vi "油动机输入合法性检查.vi"(3 "error in (no error)":errorcluster) -> (0 "error out":errorcluster, 2 "油动机名称":string)   [LabVIEW 2013]
panel:
  in  "油动机名称库":string[](array[string])
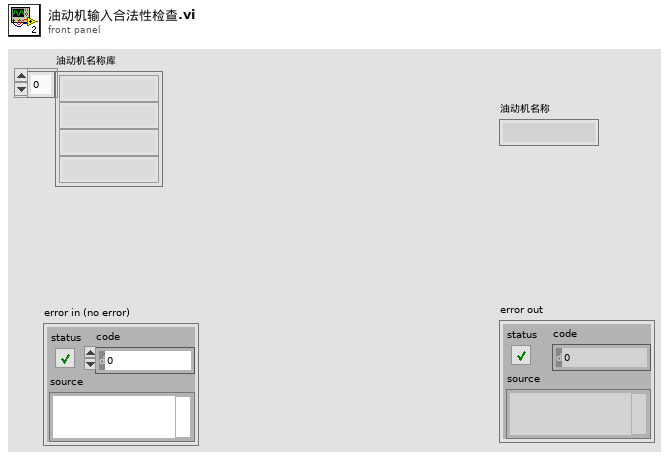
[diagram p1: front panel]
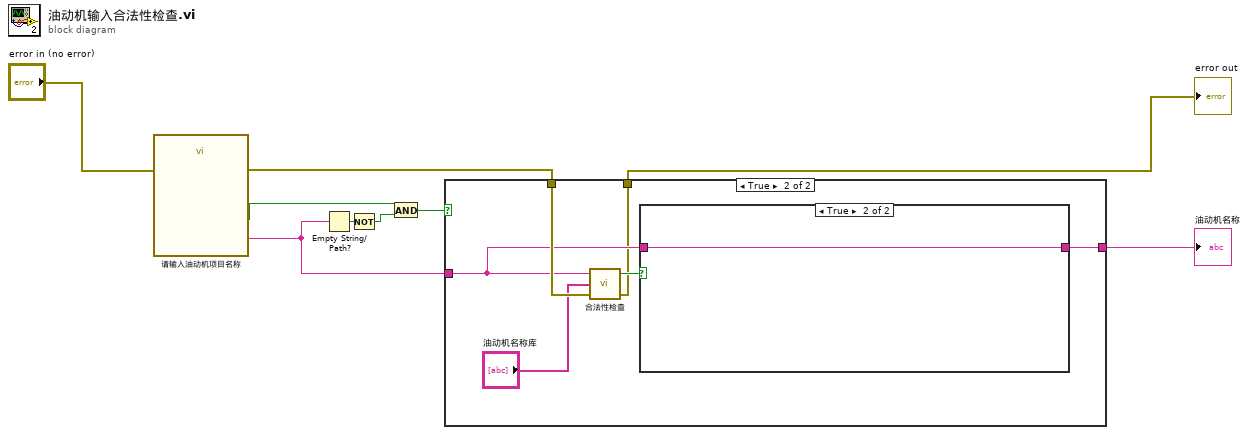
[diagram p0: block diagram]
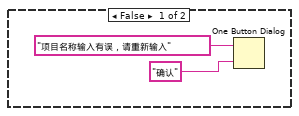
[diagram p3: hidden frame]
diagram:
  n1 = call "请输入油动机项目名称"("error in (no error)"="error in (no error)") -> ("油动机名称"=w3:string, "确认"=w7:bool, "error out"=w4:errorcluster)  [unwired: 16 in]
  n2 = Empty String/Path?(string/path=w3) -> (empty?=w9:bool)
  n3 = Not(x=w9) -> (.not. x?=w8:bool)
  n4 = And(x=w7, y=w8) -> (x .and. y?=w6:bool)
  n5 = case shown="True" w6 {
    tunnel: w4 -> [_ w15]
    tunnel: w3 -> [_ w12]
    tunnel: [_ w11] -> w2
    tunnel: [_ w10] -> w1
    frame False {
    }
    frame True {
      n6 = call "合法性检查.vi"("error in (no error)"=w15, "字符串库"="油动机名称库", "被检查字符串"=w12) -> ("error out"=w10:errorcluster, "输入有效"=w13:bool)  [unwired: 1 in]
      n7 = case shown="True" w13 {
        tunnel: w12 -> [_ w18]
        tunnel: [_ w18] -> w11
        frame False {
          n8 = One Button Dialog(message="项目名称输入有误，请重新输入", button name ("OK")="确认") -> ()  [unwired: 1 out]
        }
        frame True {
        }
      }
    }
  }
  "error out" <- w1
  "油动机名称" <- w2
